vi "Write_PLC.vi"(4 "OPC UA client refnum out":T1, 5 "error out 2":errorcluster, 6 "Direction":bool, 7 "Start_communication":bool, 8 "Relative_Motor_position":dbl) -> (0 "error out":errorcluster, 1 "Start_communication 2":bool, 2 "OPC UA client refnum out 2":T1, 3 "recommended delay":dbl)   [LabVIEW 2018]
uses:
  <vilib>/OPCUA/controls/OPC UA Client Refnum.ctl
  <vilib>/OPCUA/controls/NodeId.ctl
panel:
  out "Pulse_duration_cent":u32
  out "Pulse_duration":u32
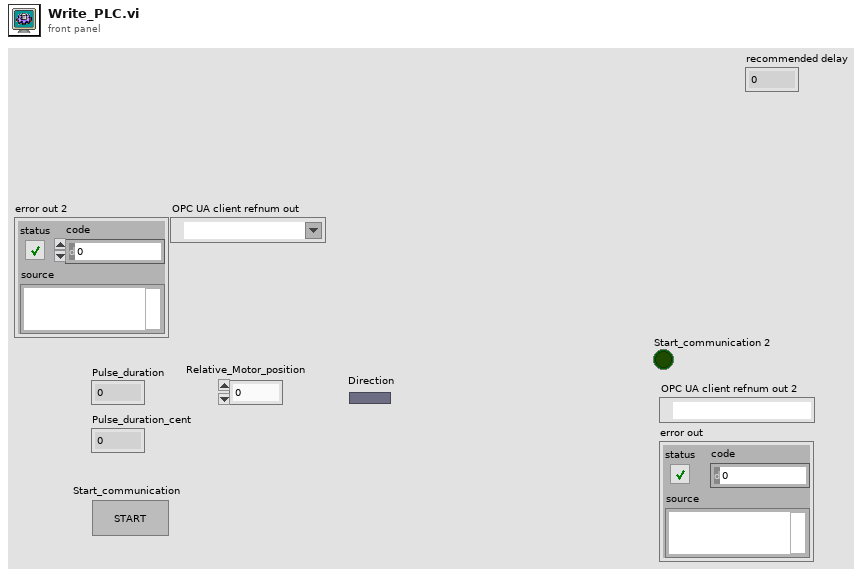
[diagram p1: front panel]
types:
  T1 = typedef "OPC UA Client Refnum.ctl" = refnum<k21>
  T2 = typedef "NodeId.ctl" = string
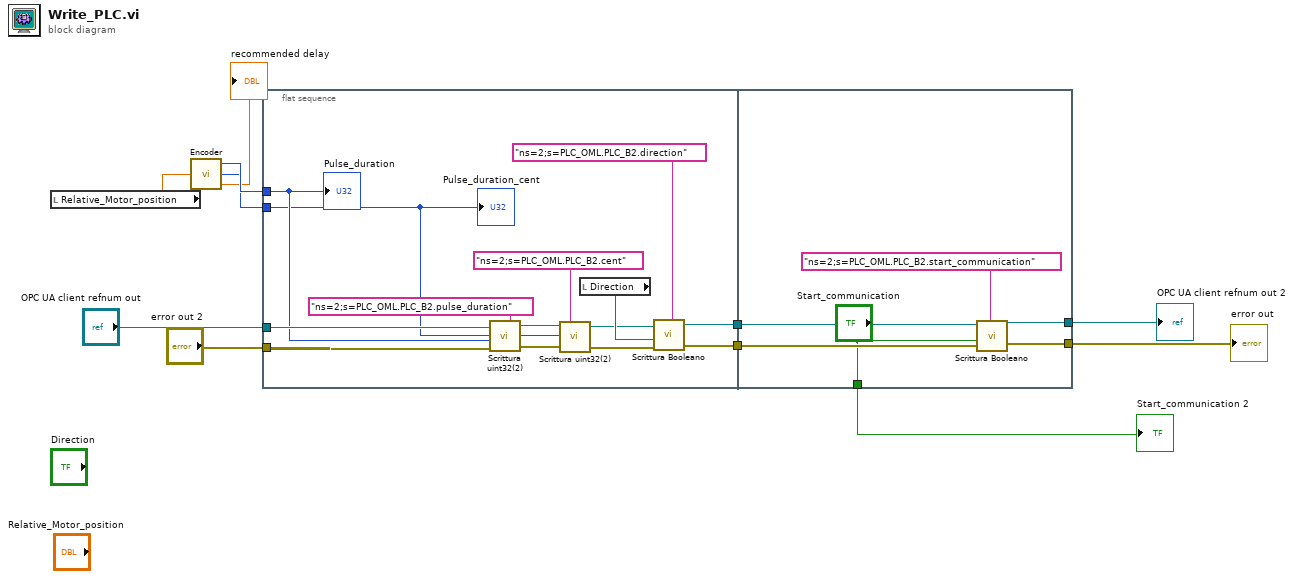
[diagram p0: block diagram]
diagram:
  n1 = local read "Relative_Motor_position"() -> (w11:dbl)
  n2 = call "Encoder.vi"("Relative_Motor_position"=w11) -> ("Pulse_duration"=w10:u32, "Pulse_duration_cent"=w9:u32, "recommended delay"=→"recommended delay":dbl)
  n3 = flat-sequence {
    tunnel: w10 -> [w15]
    tunnel: "OPC UA client refnum out" -> [w25]
    tunnel: "error out 2" -> [w24]
    tunnel: w9 -> [w13]
    tunnel: [w18] -> w8
    tunnel: [w17] -> w7
    tunnel: w8 -> [w31]
    tunnel: w7 -> [w30]
    tunnel: [w29] -> w6
    tunnel: [w28] -> w5
    tunnel: ["Start_communication"] -> w4
    frame #0 {
      n4 = call "Scrittura uint32(2).vi"("OPC UA client refnum in"=w25, "node ID"=T2 "ns=2;s=PLC_OML.PLC_B2.pulse_duration" ("Pulse_duration"), "value"=w15, "error in (no error)"=w24) -> ("OPC UA client refnum out"=w22:T1, "error out"=w23:errorcluster)  [unwired: 1 in, 1 out]
      n5 = call "Scrittura uint32(2).vi"("OPC UA client refnum in"=w22, "node ID"=T2 "ns=2;s=PLC_OML.PLC_B2.cent" ("Pulse_duration_cent"), "value"=w13, "error in (no error)"=w23) -> ("OPC UA client refnum out"=w20:T1, "error out"=w19:errorcluster)  [unwired: 1 in, 1 out]
      n6 = local read "Direction"() -> (w21:bool)
      n7 = call "Scrittura Booleano.vi"("OPC UA client refnum in"=w20, "node ID"=T2 "ns=2;s=PLC_OML.PLC_B2.direction" ("Direction"), "Value"=w21, "error in (no error)"=w19) -> ("OPC UA client refnum out"=w18:T1, "error out"=w17:errorcluster)  [unwired: 1 in, 1 out]
      "Pulse_duration" <- w15
      "Pulse_duration_cent" <- w13
    }
    frame #1 {
      n8 = call "Scrittura Booleano.vi"("OPC UA client refnum in"=w31, "node ID"=T2 "ns=2;s=PLC_OML.PLC_B2.start_communication" ("Start_comunication"), "Value"="Start_communication", "error in (no error)"=w30) -> ("OPC UA client refnum out"=w29:T1, "error out"=w28:errorcluster)  [unwired: 1 in, 1 out]
    }
  }
  "OPC UA client refnum out 2" <- w6
  "error out" <- w5
  "Start_communication 2" <- w4
